vi "Hab Driver Controller.vi"(8 "error in":errorcluster) -> ()   [LabVIEW 2018]
doc: "This VI executes continuously carrying out the current operation and responding to updates or new operations. It will often contain the timing or control code that is difficult to place directly in TeleOp. This VI generally opens all sensors and motors and isolates the rest of the robot code from knowing how the operations are carried out."
uses:
  <vilib>/Rock Robotics/WPI/Framework/Completion Status.ctl
  Hab Driver Setpoints.ctl
  Hab Driver Operations.ctl
  <vilib>/Rock Robotics/WPI/ThirdParty/Phoenix-LabVIEW/Motor Controller/Controls/CTRE_Phoenix_MotorControl_ControlMode.ctl
  <vilib>/Rock Robotics/Network Tables/NT Read Number.vi
  <vilib>/Rock Robotics/Network Tables/NT Write Boolean.vi
panel:
  in  "Interactive Values":T1
  out "Current\nCmd":string
  in  "Buttons":cluster{"Execute Cmd":bool, "Abort Cmd":bool}
  out "Command Timing":cluster{"Start Time (ms)":u32, "Iterations":i32}
  out "Status":T3
  # "Tip: It may be helpful to observe inputs and sensor values.\nYou may also want to display tuning or debugging controls."
  # "Interactive Command: You may fill in the settings for a command\nand schedule it with the Execute button. You can observe and abort\nany command while fine tuning the code for the controller."
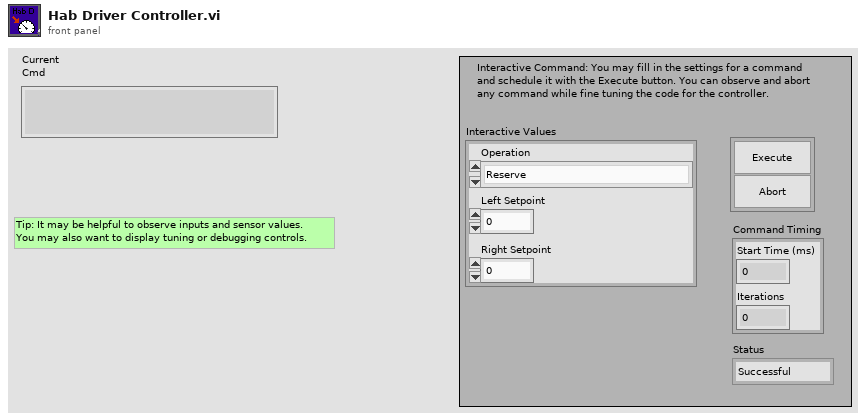
[diagram p1: front panel]
types:
  T1 = typedef "Hab Driver Setpoints.ctl" = cluster{"Operation":T2, "Left Setpoint":dbl, "Right Setpoint":dbl}
  T2 = typedef "Hab Driver Operations.ctl" = enum16{"Reserve", "Read Current", "Immediate", "Emma: Drive around with the extendo wheels"}
  T3 = typedef "Completion Status.ctl" = enum16{"Successful", "Aborted", "Incomplete"}
  T4 = typedef "WPI_MotorControlDeviceRef.ctl" = cluster{"DeviceStatus":errorcluster, "Type":T5, "PWM":cluster{"PWM Channel":T6, "DeadBand":T7}, "CAN":cluster{"Device Number":u8, "SetOutput VI Ref":variant, "GetOutput VI Ref":variant, "Enable VI Ref":variant, "Disable VI Ref":variant, "Data":variant}, "Invert":bool, "DIO PWM":cluster{"PWM \"Enable\" Channel":T6, "DIOChannel":T8, "PWM Rate":dbl}}
  T5 = typedef "WPI_MotorControlType.ctl" = enum16{"PWM", "CAN", "DIO PWM"}
  T6 = typedef "FPGA_DIOPWMChannel.ctl" = enum8{"PWM 0", "PWM 1", "PWM 2", "PWM 3", "PWM 4", "PWM 5", "PWM 6", "PWM 7", "PWM 8", "PWM 9", "PWM MXP 0", "PWM MXP 1", "PWM MXP 2", "PWM MXP 3", "PWM MXP 4", "PWM MXP 5", "PWM MXP 6", "PWM MXP 7", "PWM MXP 8", "PWM MXP 9", "Invalid"}
  T7 = typedef "WPI_PWMDeadband.ctl" = cluster{"Name":string, "maxPositivePwm":i32, "minPositivePwm":i32, "centerPwm":i32, "maxNegativePwm":i32, "minNegativePwm":i32, "angularRange":u16}
  T8 = typedef "FPGA_DIOChannel.ctl" = enum8{"DIO 0", "DIO 1", "DIO 2", "DIO 3", "DIO 4", "DIO 5", "DIO 6", "DIO 7", "DIO 8", "DIO 9", "DIO MXP 0", "DIO MXP 1", "DIO MXP 2", "DIO MXP 3", "DIO MXP 4", "DIO MXP 5", "DIO MXP 6", "DIO MXP 7", "DIO MXP 8", "DIO MXP 9", "DIO MXP 10", "DIO MXP 11", "DIO MXP 12", "DIO MXP 13", "DIO MXP 14", "DIO MXP 15", "SPI Port CS1", "SPI Port CS2", "SPI Port CS3", "SPI Port MISO", "SPI Port MOSI", "Invalid"}
  T9 = typedef "Command Status Info.ctl" = cluster{"Name":string, "Status":T3, "notifier out":T10}
  T10 = typedef "Completion Notifier.ctl" = refnum<notifier>
  T11 = cluster{"Current Command":T1, "Command Timing":cluster{"Start Time (ms)":u32, "Iterations":i32}, "Command Arguments":cluster{"Command Info":T9, "Description":string, "Default Command":T1, "queue out":refnum<queue>, "Subsystem Name":string}}
  T12 = typedef "CTRE_Phoenix_MotorControl_ControlMode.ctl" = u16
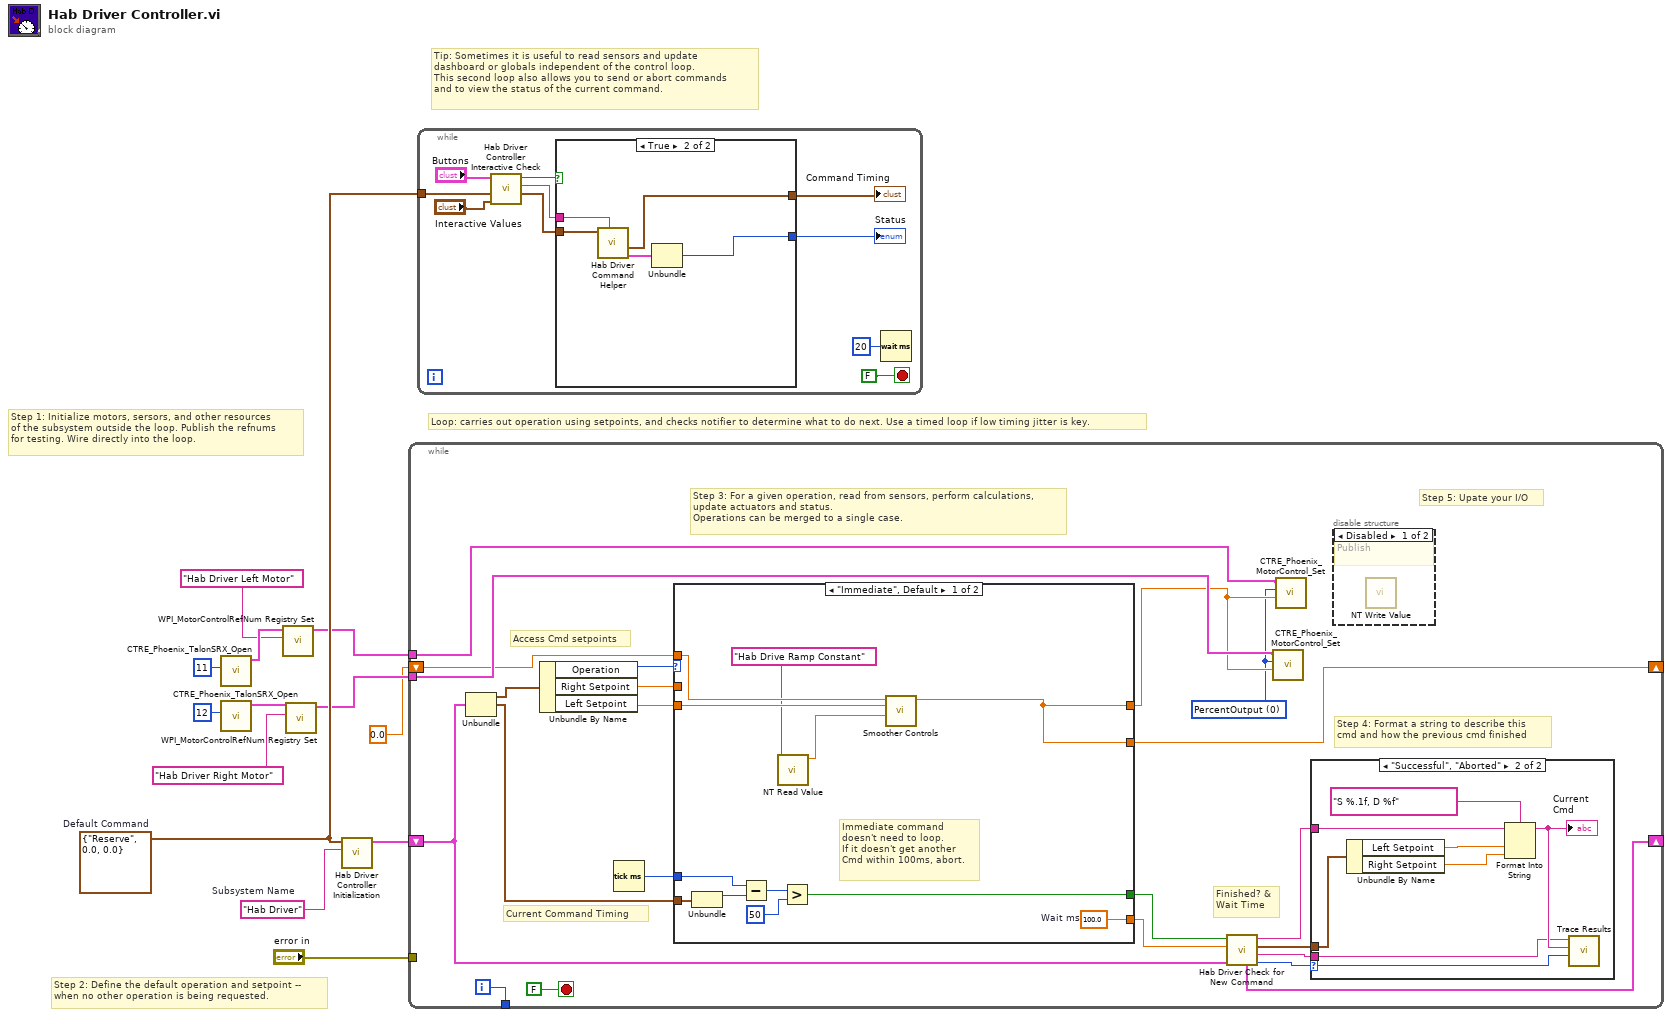
[diagram p0: block diagram]
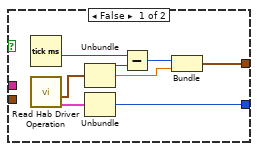
[diagram p2: hidden frame]
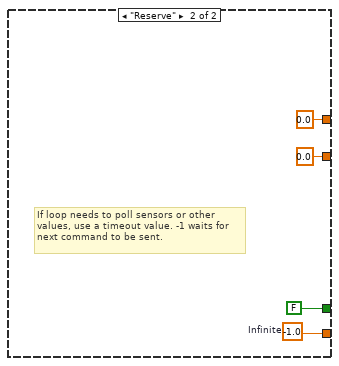
[diagram p5: hidden frame]
diagram:
  w10 = T1 {"Operation"=enum."Reserve", "Left Setpoint"=0.0, "Right Setpoint"=0.0}  # Default Command
  w11 = "Hab Driver"  # Subsystem Name
  # "Tip: Sometimes it is useful to read sensors and update\ndashboard or globals independent of the control loop.\nThis second loop also allows you to send or abort commands\nand to view the status of the current command."
  # "Step 2: Define the default operation and setpoint --\nwhen no other operation is being requested."
  # "Step 1: Initialize motors, sersors, and other resources\nof the subsystem outside the loop. Publish the refnums\nfor testing. Wire directly into the loop."
  # "Loop: carries out operation using setpoints, and checks notifier to determine what to do next. Use a timed loop if low timing jitter is key."
  n1 = call <vilib>:"CTRE_Phoenix_TalonSRX_Open.vi"("Device Number"=u8 11) -> ("CAN Talon SRX Ref"=w7:T4)  [unwired: 9 in, 1 out]
  n2 = call <vilib>:"CTRE_Phoenix_TalonSRX_Open.vi"("Device Number"=u8 12) -> ("CAN Talon SRX Ref"=w4:T4)  [unwired: 9 in, 1 out]
  n3 = call <vilib>:"WPI_MotorControlRefNum Registry Set.vi"("refnum name"="Hab Driver Left Motor", "MotorControlDevRef"=w7) -> ("MotorControlDevRef"=w6:T4)  [unwired: 8 in, 1 out]
  n4 = call <vilib>:"WPI_MotorControlRefNum Registry Set.vi"("refnum name"="Hab Driver Right Motor", "MotorControlDevRef"=w4) -> ("MotorControlDevRef"=w2:T4)  [unwired: 8 in, 1 out]
  n5 = call "Hab Driver Controller Initialization.vi"("Subsystem Name"=w11, "Default Command"=w10) -> ("Current Command"=w12:T11)  [unwired: 9 in]
  n6 = while {
    shift-right: [w27] -> _
    shift-left: w12 -> [w20]
    tunnel: [w34] -> _
    tunnel: "error in" -> [_]
    tunnel: w6 -> [w19]
    tunnel: w2 -> [w18]
    shift-right: [w15] -> _
    shift-left: 0.0 -> [w14]
    i -> [w34]
    stop <- FALSE stop-if-true
    w16 = T12 0 items=["PercentOutput"=0, "Position"=1, "Velocity"=2, "Current"=3, "Follower"=5, "MotionProfile"=6, "MotionMagic"=7, "MotionProfileArc"=10, "Disabled"=15] ("Control Mode")
    # "Step 5: Upate your I/O"
    # "Step 4: Format a string to describe this\ncmd and how the previous cmd finished"
    # "Current Command Timing"
    # "Access Cmd setpoints"
    # "Finished? &\nWait Time"
    # "Step 3: For a given operation, read from sensors, perform calculations,\nupdate actuators and status.\nOperations can be merged to a single case."
    n7 = Unbundle(w20) -> ("Current Command"=w33:T1, "Command Timing"=w29:cluster{"Start Time (ms)":u32, "Iterations":i32})  [unwired: 1 out]
    n8 = Unbundle By Name(w33) -> ("Operation"=w32:T2, "Right Setpoint"=w31:dbl, "Left Setpoint"=w28:dbl)
    n9 = Tick Count (ms)() -> (millisecond timer value=w30:u32)
    n10 = case shown="\"Immediate\", Default" w32 {
      tunnel: [w55 w59] -> w25
      tunnel: [w49 FALSE ("ignore previous (F)")] -> w26
      tunnel: w29 -> [w51 _]
      tunnel: w31 -> [_ _]
      tunnel: w30 -> [w50 _]
      tunnel: w28 -> [w48 _]
      tunnel: [w46 0.0 ("Setpoint")] -> w17
      tunnel: [w46 0.0 ("Motor Setpoint")] -> w15
      tunnel: w14 -> [w47 _]
      frame "Immediate", Default {
        w55 = 100.0  # Wait ms
        # "Immediate command\ndoesn't need to loop.\nIf it doesn't get another\nCmd within 100ms, abort."
        n11 = Unbundle(w51) -> ("Start Time (ms)"=w54:u32)  [unwired: 1 out]
        n12 = Subtract(x=w50, y=w54) -> (x-y=w53:u32)
        n13 = call-poly <vilib>:"NT Read Value.vi"("Name"="Hab Drive Ramp Constant") -> ("Numeric"=w45:dbl)  [unwired: 9 in, 1 out]
        n14 = Greater?(x=w53, y=u8 50 ("Left Motor")) -> (0:w49:bool)
        n15 = call "Smoother Controls.vi"("Proportional Constant"=w45, "New Input"=w48, "Previous Value"=w47) -> ("Motor Setpoint"=w46:dbl)  [unwired: 8 in]
      }
      frame "Reserve" {
        w59 = -1.0  # Infinite
        # "If loop needs to poll sensors or other\nvalues, use a timeout value. -1 waits for\nnext command to be sent."
      }
    }
    n16 = call "Hab Driver Check for New Command.vi"("Current Command"=w20, "Wait time (ms)"=w25, "Finished?"=w26) -> ("Completion"=w21:T3, "Subsystem Name"=w22:string, "Current Command"=w23:T1, "Initial Trace String"=w24:string, "NextCommand"=w27:T11)  [unwired: 4 in]
    n17 = call <vilib>:"CTRE_Phoenix_MotorControl_Set.vi"("Output"=w17, "Control Mode"=w16, "PhoenixMotorControlDevRef"=w18) -> ()  [unwired: 7 in, 2 out]
    n18 = call <vilib>:"CTRE_Phoenix_MotorControl_Set.vi"("Output"=w17, "Control Mode"=w16, "PhoenixMotorControlDevRef"=w19) -> ()  [unwired: 7 in, 2 out]
    n19 = case shown="\"Successful\", \"Aborted\"" w21 {
      selector: w21 -> [_ w43]
      tunnel: w24 -> [_ w39]
      tunnel: w23 -> [_ w40]
      tunnel: w22 -> [_ w36]
      frame "Incomplete", Default {
        # "Continuing current command"
      }
      frame "Successful", "Aborted" {
        # "Report and setup for next command"
        n20 = Unbundle By Name(w40) -> ("Left Setpoint"=w42:dbl, "Right Setpoint"=w37:dbl)
        n21 = Format Into String(format string="S %.1f, D %f", initial string=w39, w42, w37) -> (resulting string=w38:string)  [unwired: 1 in, 1 out]
        "Current\nCmd" <- w38
        n22 = call <vilib>:"Trace Results.vi"("Status of previous command"=w43, "Description"=w38, "Subsystem"=w36) -> ()  [unwired: 9 in]
      }
    }
    n23 = disable-structure shown="Disabled" {
      frame Disabled {
        # "Publish"
        n24 = call-poly <vilib>:"NT Write Value.vi"() -> ()  [unwired: 11 in, 1 out]
      }
      frame Enabled {
      }
    }
  }
  n25 = while {
    tunnel: w10 -> [w66]
    stop <- FALSE stop-if-true
    n26 = call "Hab Driver Controller Interactive Check.vi"("Interactive Command in"="Interactive Values", "Default Command"=w66, "Buttons"="Buttons") -> ("Interactive Command out"=w63:T1, "Trace String"=w64:string, "Schedule"=w65:bool)  [unwired: 6 in]
    n27 = case shown="True" w65 {
      tunnel: [w77 w82] -> w62
      tunnel: w63 -> [_ w80]
      tunnel: [w73 w78] -> w61
      tunnel: w64 -> [_ w81]
      frame False {
        n28 = Tick Count (ms)() -> (millisecond timer value=w72:u32)
        n29 = call "Read Hab Driver Operation.vi"() -> ("Command Info"=w70:T9, "SubSystem Data"=w71:T1)  [unwired: 9 in, 1 out]
        n30 = Unbundle(w71) -> ("Operation"=w76:T2, "Left Setpoint"=w74:dbl)  [unwired: 1 out]
        n31 = Unbundle(w70) -> ("Status"=w77:T3)  [unwired: 2 out]
        n32 = Subtract(x=w72, y=w76) -> (x-y=w75:u32)
        n33 = Bundle(w75, "Left Setpoint"=w74) -> (w73:cluster{u32, "Left Setpoint":dbl})  [unwired: 1 in]
      }
      frame True {
        n34 = call "Hab Driver Command Helper.vi"("Description"=w81, "SubSystem Data"=w80) -> ("Command Info Out"=w79:T9, "Command Timing"=w78:cluster{"Start Time (ms)":u32, "Iterations":i32})  [unwired: 7 in, 1 out]
        n35 = Unbundle(w79) -> ("Status"=w82:T3)  [unwired: 2 out]
      }
    }
    "Status" <- w62
    "Command Timing" <- w61
    n36 = Wait (ms)(milliseconds to wait=u32 20) -> ()  [unwired: 1 out]
  }
